vi "Get_DSC_Vals.vi"(8 "Machine":string, 9 "Shared Variable Control":refnum<k21>, 10 "Name":string, 11 "Authorization Header":T1[](array[typedef])) -> ()   [LabVIEW 2016]
uses:
  <vilib>/addons/_JKI.lib/REST Client/classes/REST Client/HTTP Header.ctl
  <vilib>/LVH/i3 JSON/JSON Parsing/Get Object Parameter Files/Get Object Parameter - Object.vi
  <vilib>/LVH/i3 JSON/JSON Parsing/Get Object Parameter Files/Get Object Parameter - String.vi
  <vilib>/addons/_JKI.lib/REST Client/classes/REST Client/REST Client.lvclass
  <vilib>/addons/_JKI.lib/Serialization/JSON/JKI JSON Serialization.lvlib
  <vilib>/LVH/i3 JSON/i3-json.lvlib
panel:
  in  "OK":bool
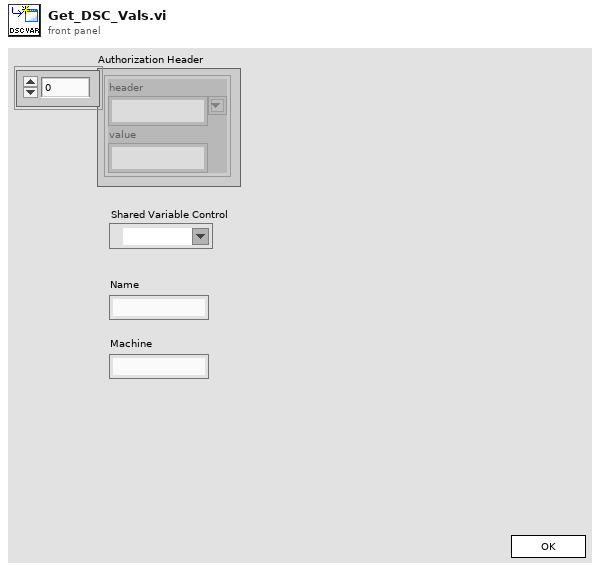
[diagram p1: front panel]
types:
  T1 = typedef "REST Client.lvlib/REST Client.lvclass/HTTP Header.ctl" = cluster{"header":string, "value":string}
  T2 = enum32{"Invalid", "Standard", "Closed", "Hidden", "Minimized", "Maximized"}
  T3 = enum32{"invalid app kind", "Development System", "Run Time System", "Student Edition", "Embedded LabVIEW", "Evaluation", "Custom"}
  T4 = cluster{"Core":cluster{"Current VI Reference":refnum<vi>, "Close Panel on Exit?":bool}, "New Reference":string, "Array of DSC References":cluster{string, string}[], "Authorization Header":T1[], "GID":string, "Name":string, "trimmed string":string, "Section GID":string}
  T5 = cluster{"Current VI Reference":refnum<vi>, "Close Panel on Exit?":bool}
  T6 = cluster{"data":cluster{"id":i32, "gid":string, "name":string, "resource_type":string}[]}
  T7 = cluster{"id":i32, "gid":string, "name":string, "resource_type":string}[]
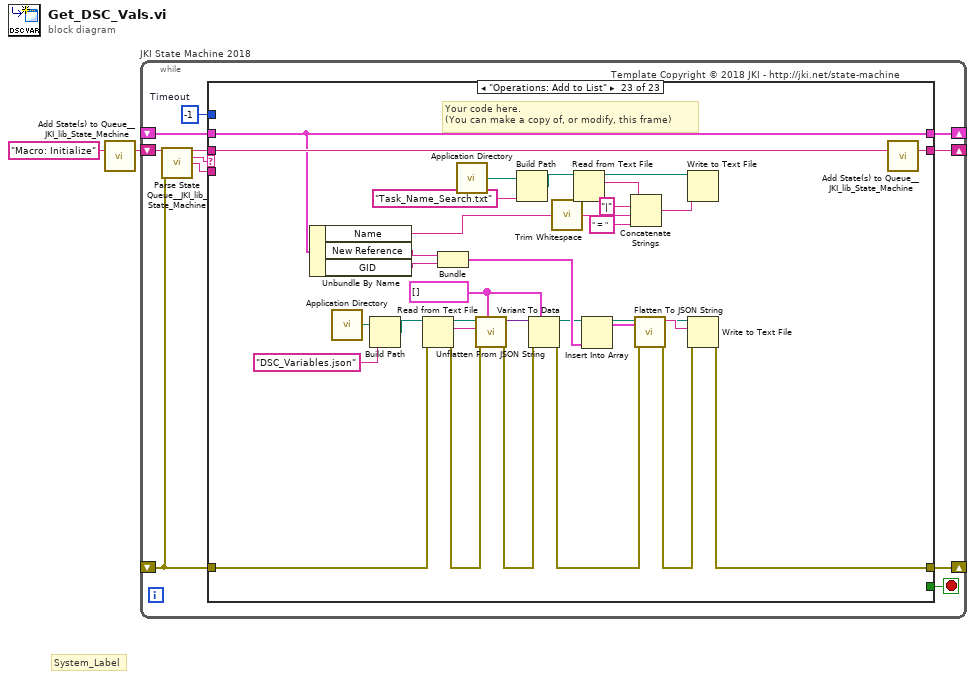
[diagram p0: block diagram]
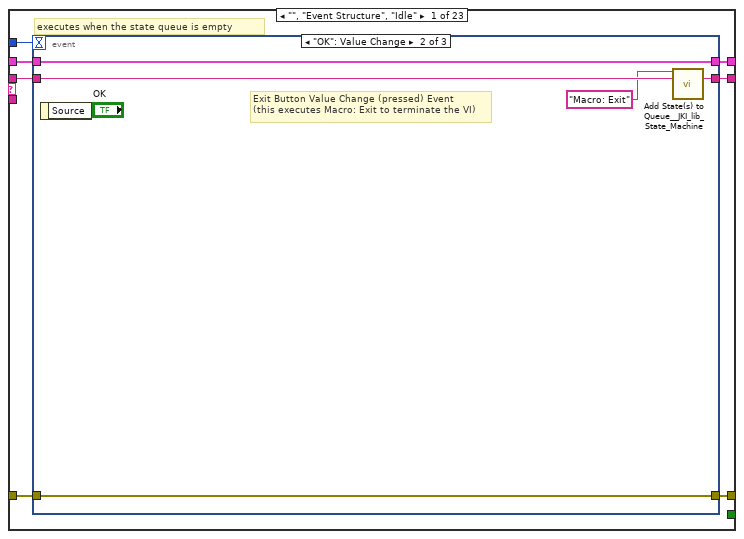
[diagram p2: hidden frame]
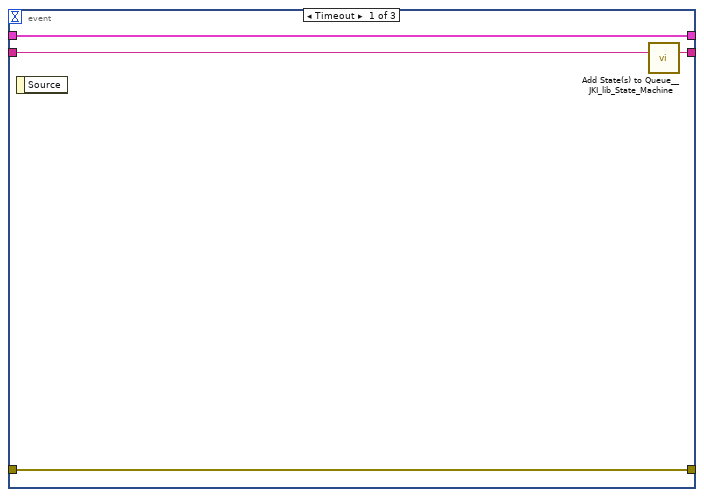
[diagram p3: hidden frame]
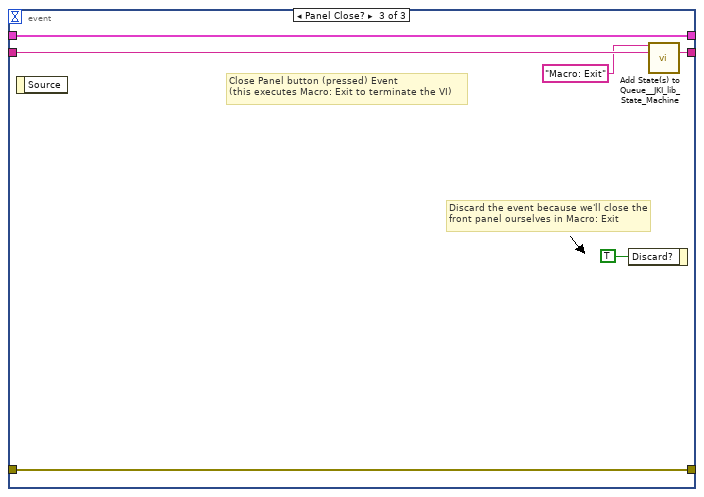
[diagram p4: hidden frame]
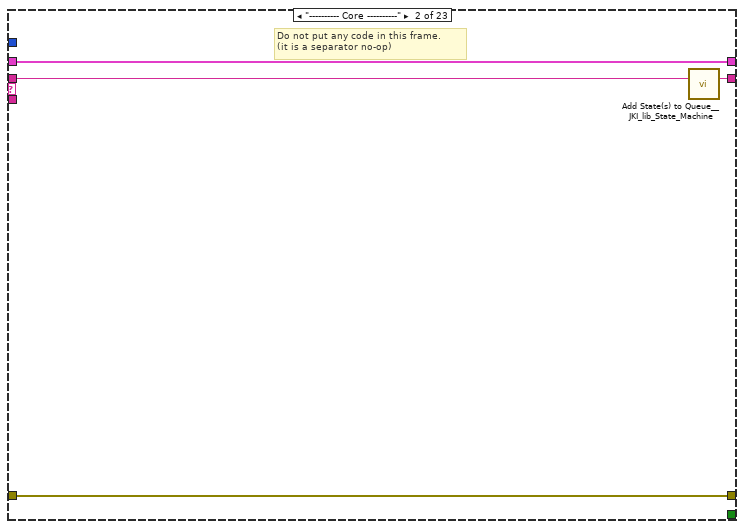
[diagram p5: hidden frame]
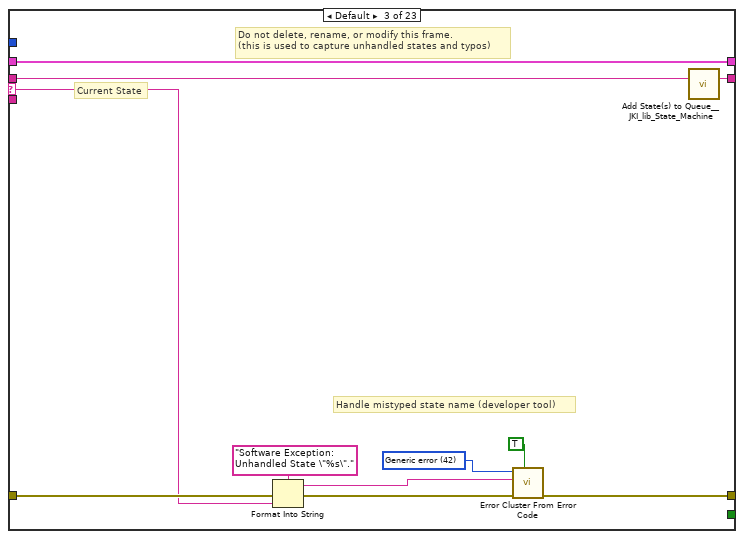
[diagram p6: hidden frame]
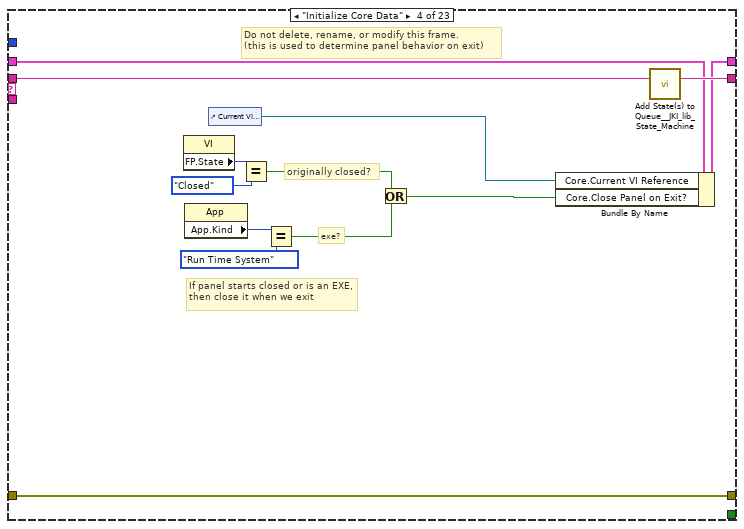
[diagram p7: hidden frame]
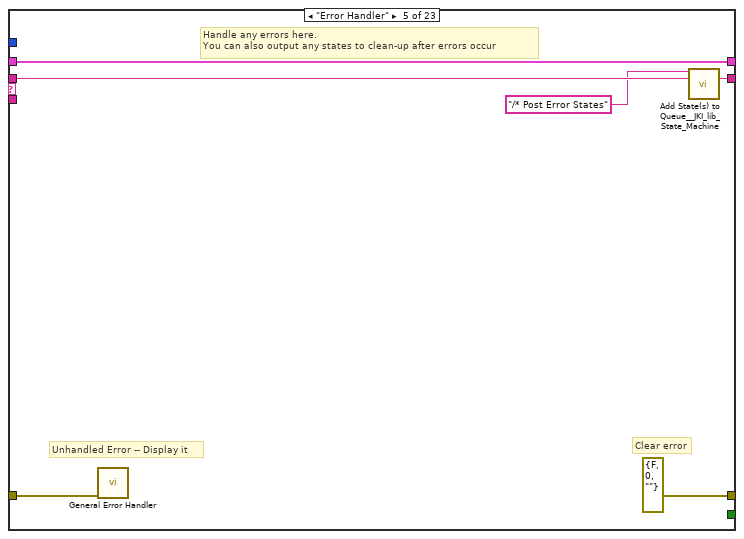
[diagram p8: hidden frame]
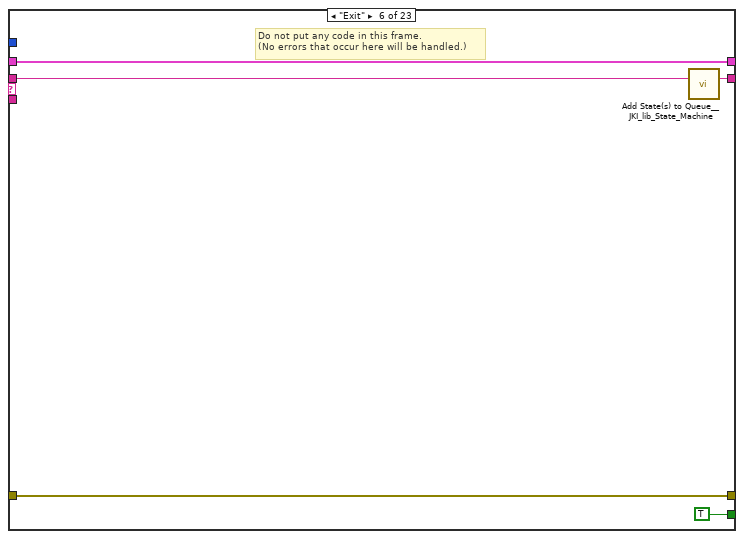
[diagram p9: hidden frame]
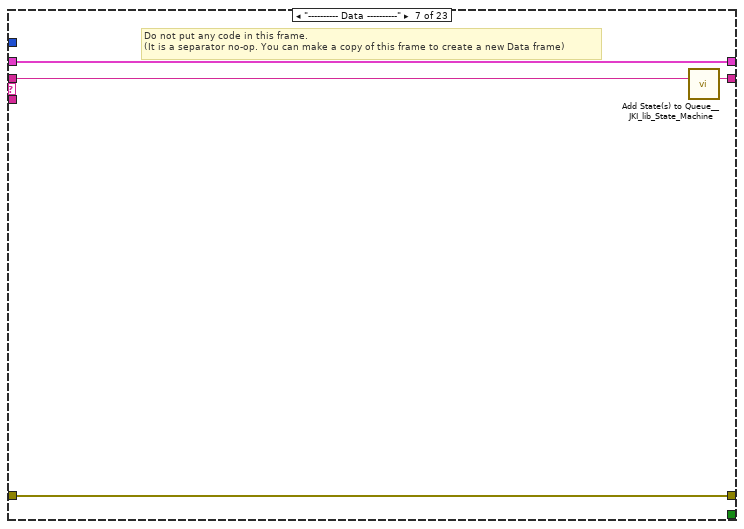
[diagram p10: hidden frame]
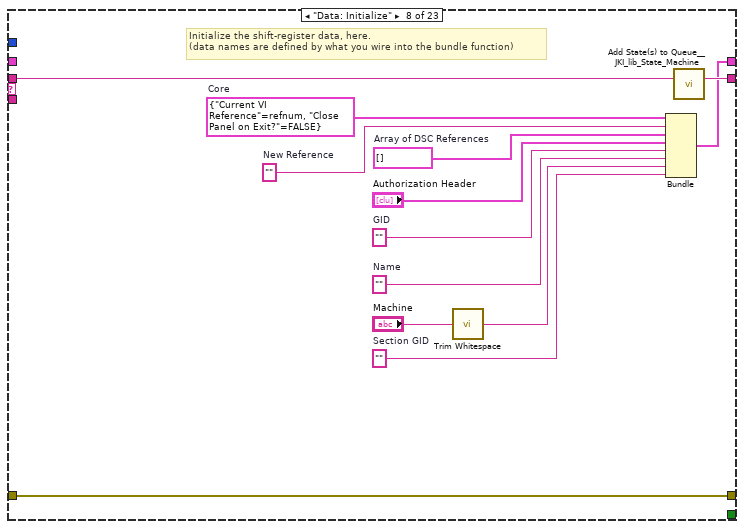
[diagram p11: hidden frame]
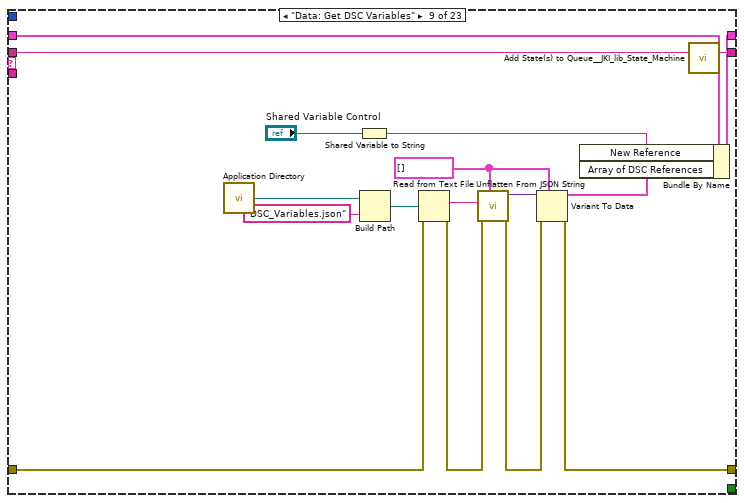
[diagram p12: hidden frame]
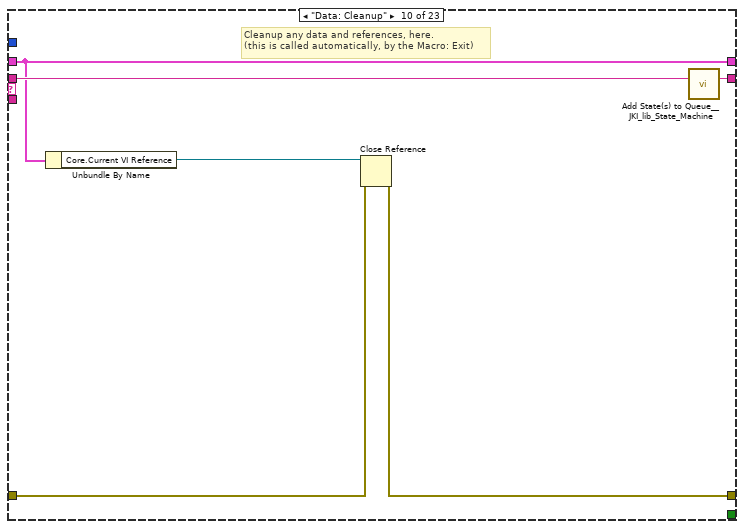
[diagram p13: hidden frame]
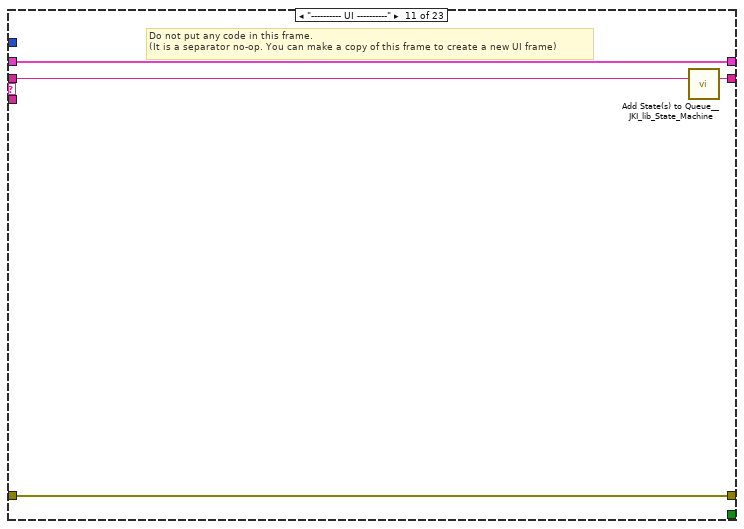
[diagram p14: hidden frame]
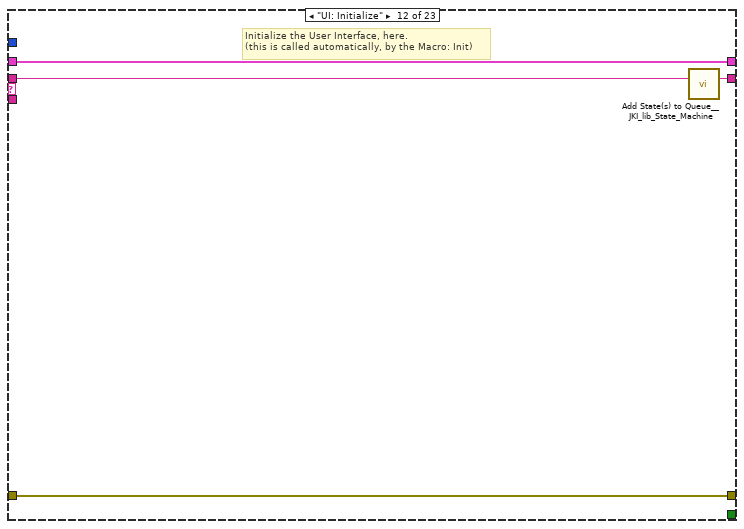
[diagram p15: hidden frame]
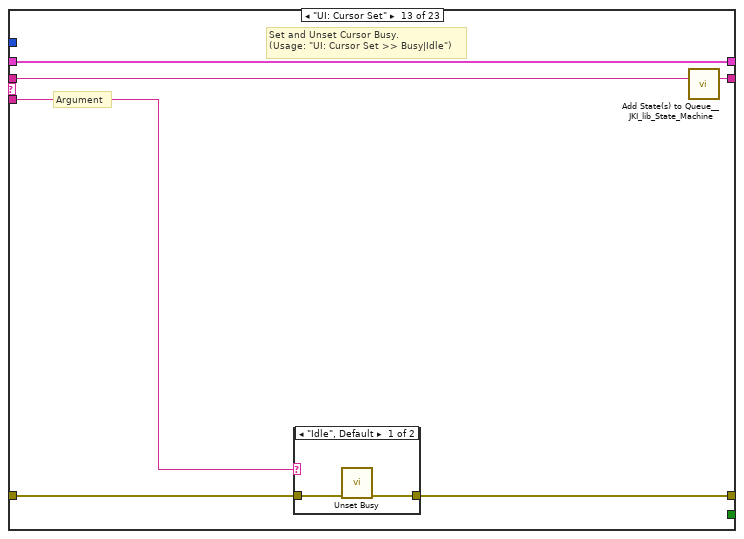
[diagram p16: hidden frame]
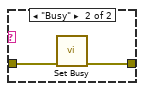
[diagram p17: hidden frame]
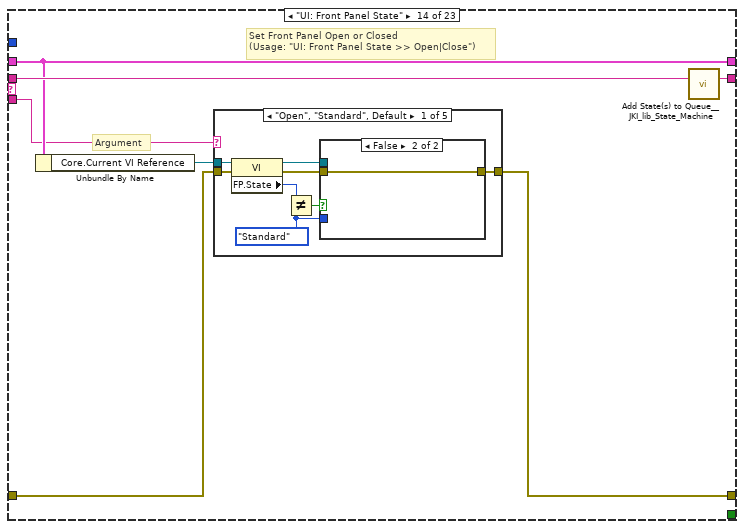
[diagram p18: hidden frame]
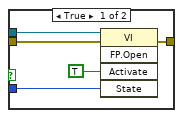
[diagram p19: hidden frame]
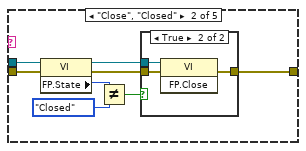
[diagram p20: hidden frame]
diagram:
  # "System_Label"
  n1 = call <vilib>:"Add State(s) to Queue__JKI_lib_State_Machine.vi"("State(s) in (\"\")"="Macro: Initialize") -> ("States Out"=w2:string)  [unwired: 14 in]
  n2 = while "JKI State Machine 2018" {
    shift-right: [w6] -> _
    shift-left: _ -> [w5]
    shift-right: [w9] -> _
    shift-left: _ -> [w3]
    shift-right: [w8] -> _
    shift-left: w2 -> [w10]
    stop <- w7 stop-if-true
    w4 = -1  # Timeout
    # "Template Copyright © 2018 JKI - http://jki.net/state-machine"
    n3 = call <vilib>:"Parse State Queue__JKI_lib_State_Machine.vi"("State Queue"=w10, "Error In (no error)"=w3) -> ("Remaining States"=w12:string, "Current State"=w13:string, "Arguments"=w11:string)  [unwired: 11 in]
    n4 = case shown="\"Operations: Add to List\"" w13 {
      selector: w13 -> [_ _ w40 _ _ _ _ _ _ _ _ _ _ _ _ _ _ _ _ _ _ _ _]
      tunnel: w12 -> [w20 w39 w44 w63 w69 w74 w78 w91 w108 w114 w118 w122 w128 w139 w208 w213 w223 w227 w237 w269 w307 w333 w363]
      tunnel: w11 -> [_ _ _ _ _ _ _ _ _ _ _ _ w123 w133 _ _ _ _ _ _ _ _ _]
      tunnel: w5 -> [w18 w36 w42 w56 w66 w72 w75 _ w105 w109 w115 w120 w126 w135 w205 w210 w220 w224 w234 w246 w301 w324 w361]
      tunnel: [w17 w37 w46 w60 errorcluster {"status"=FALSE, "code"=0, "source"=""} ("error out") w71 w76 w88 w96 w110 w116 w119 w124 w136 w206 w211 w221 w225 w235 w255 w296 w316 w357] -> w9
      tunnel: w3 -> [w16 w37 w45 w60 w65 w71 w76 w88 w95 w111 w116 w119 w125 w137 w206 w211 w221 w225 w235 w260 w299 w322 w358]
      tunnel: [w19 w38 w43 w62 w68 w73 w77 w90 w107 w113 w117 w121 w127 w138 w207 w212 w222 w226 w236 w268 w306 w332 w362] -> w8
      tunnel: [_ _ _ _ _ TRUE _ _ _ _ _ _ _ _ _ _ _ _ _ _ _ _ _] -> w7
      tunnel: [w15 w36 w42 w61 w66 w72 w75 w89 w104 w109 w115 w120 w126 w135 w205 w210 w220 w224 w234 w245 w300 w323 w361] -> w6
      tunnel: w4 -> [w14 _ _ _ _ _ _ _ _ _ _ _ _ _ _ _ _ _ _ _ _ _ _]
      frame "", "Event Structure", "Idle" {
        # "executes when the state queue is empty"
        n5 = event shown="[1] \"OK\": Value Change" {
          selector: _ -> [_ _ _]
          dyn-events: _ -> [_ _ _]
          timeout: w14 -> [_ _ _]
          tunnel: w20 -> [w24 w29 w35]
          tunnel: [w23 w28 w34] -> w19
          tunnel: w18 -> [w21 w26 w32]
          tunnel: [w22 w27 w33] -> w17
          tunnel: w16 -> [w22 w27 w33]
          tunnel: [w21 w26 w32] -> w15
          event Timeout {
            n6 = event-data() -> ()  [unwired: 1 in, 1 out]
            n7 = call <vilib>:"Add State(s) to Queue__JKI_lib_State_Machine.vi"("State(s) in (\"\")"=w24) -> ("States Out"=w23:string)  [unwired: 14 in]
          }
          event "OK": Value Change {
            # "Exit Button Value Change (pressed) Event\n(this executes Macro: Exit to terminate the VI)"
            n8 = event-data() -> ()  [unwired: 1 in, 1 out]
            n9 = call <vilib>:"Add State(s) to Queue__JKI_lib_State_Machine.vi"("State(s) in Front (\"\")"="Macro: Exit", "State(s) in (\"\")"=w29) -> ("States Out"=w28:string)  [unwired: 13 in]
          }
          event Panel Close? {
            # "Discard the event because we'll close the front panel ourselves in Macro: Exit"
            # "Close Panel button (pressed) Event\n(this executes Macro: Exit to terminate the VI)"
            n10 = event-data() -> ()  [unwired: 1 in, 1 out]
            n11 = event-data("Discard?"=TRUE) -> ()  [unwired: 1 in, 1 out]
            n12 = call <vilib>:"Add State(s) to Queue__JKI_lib_State_Machine.vi"("State(s) in Front (\"\")"="Macro: Exit", "State(s) in (\"\")"=w35) -> ("States Out"=w34:string)  [unwired: 13 in]
          }
        }
      }
      frame "---------- Core ----------" {
        # "Do not put any code in this frame.\n(it is a separator no-op)"
        n13 = call <vilib>:"Add State(s) to Queue__JKI_lib_State_Machine.vi"("State(s) in (\"\")"=w39) -> ("States Out"=w38:string)  [unwired: 14 in]
      }
      frame Default {
        w49 = 42 items=["No error", "Argument error", "Memory is full", "Out of zone", "End of file", "File already open", "Generic file I/O error", "File not found", "File permission error", "Disk is full", "Duplicate path", "Too many files open", "System feature not enabled", "Resource file not found", "Cannot add resource", "Resource not found", "Image not found", "Image memory error", "Pen does not exist", "Config type invalid", "Config token not found", "Config parse error", "Config memory error", "Bad external code format", "Bad external code offset", "External code not present", "Null window", "Destroy window error", "Null menu", "Print aborted", "Bad print record", "Print driver error", "Windows error during printing", "Memory error during printing", "Print dialog error", "Generic print error", "Invalid device refnum", "Device not found", "Device parameter error", "Device unit error", "Cannot open device", "Device call aborted", "Generic error", "Cancelled by user", "Object ID too low", "Object ID too high", "Object not in heap", "Unknown heap", "Unknown object (invalid DefProc)", "Unknown object (DefProc not in table)", "Message out of range", "Invalid (null) method", "Unknown message", "Manager call not supported", "Bad address", "Network operation in progress", "Network operation timed out", "Connection is busy", "Network attribute not supported", "Network error", "Address in use", "System out of memory", "Connection aborted", "Connection refused", "Not connected", "Already connected", "Connection closed", "Initialization error (interapplication manager)", "Bad occurrence", "Wait on unbound occurrence handler", "Occurrence queue overflow", "Datalog type conflict", "Unused", "Unrecognized type (interapplication manager)", "Memory corrupt", "Failed to make temporary DLL", "Old CIN version", "Drag socket not found", "Failed to load drop-object", "Failed to register OLE object", "Failed to release OLE object", "Format specifier type mismatch", "Unknown format specifier", "Too few format specifiers", "Too many format specifiers", "Scan failed", "Newer CIN version", "Error converting to variant", "Runtime menu error", "Password tampered", "Variant attribute not found", "Incompatible variant data type", "Event data is not available", "Event Store is not present", "Occurrence is not found", "Event Queue is not created", "Event info is not available", "Refnum passed is NULL", "Error retrieving Class GUID", "Error retrieving CoClass GUID", "Error retrieving TypeLib GUID.", "Bad built application magic bytes.", "Specific driver is different from the specific driver associated with the Logical Name.", "There is no session opened to the class driver.", "Max Error", "MAX - Error with config objects", "MAX - Error loading configuration", "MAX - Group not supported"]
        # "Current State"
        # "Do not delete, rename, or modify this frame.\n(this is used to capture unhandled states and typos)"
        # "Handle mistyped state name (developer tool)"
        n14 = Format Into String(format string="Software Exception: Unhandled State \"%s\"." ("message"), error in=w45, w40) -> (resulting string=w48:string, error out=w47:errorcluster)  [unwired: 1 in]
        n15 = call <vilib>:"Error Cluster From Error Code.vi"("show call chain? (False)"=TRUE, "error in (no error)"=w47, "error message (\"\")"=w48, "error code (0)"=w49) -> ("error out"=w46:errorcluster)  [unwired: 5 in]
        n16 = call <vilib>:"Add State(s) to Queue__JKI_lib_State_Machine.vi"("State(s) in (\"\")"=w44) -> ("States Out"=w43:string)  [unwired: 14 in]
      }
      frame "Initialize Core Data" {
        # "Do not delete, rename, or modify this frame.\n(this is used to determine panel behavior on exit)"
        # "originally closed?"
        # "exe?"
        # "If panel starts closed or is an EXE, then close it when we exit"
        n17 = property class="VI"() -> ("FP.State"=w53:T2)  [unwired: 2 in, 2 out]
        n18 = property class="App"() -> ("App.Kind"=w59:T3)  [unwired: 2 in, 2 out]
        n19 = control-ref of="Current VI Reference"() -> (w54:refnum<vi>)
        n20 = Equal?(x=w53, y=T2."Closed" ("Front Panel Window:State")) -> (x = y?=w51:bool)
        n21 = Equal?(x=w59, y=T3."Run Time System" ("Application:Kind")) -> (x = y?=w57:bool)
        n22 = Or(x=w51, y=w57) -> (x .or. y?=w55:bool)
        n23 = Bundle By Name(cluster=w56, "Core.Current VI Reference"=w54, "Core.Close Panel on Exit?"=w55) -> (w61:T4)
        n24 = call <vilib>:"Add State(s) to Queue__JKI_lib_State_Machine.vi"("State(s) in (\"\")"=w63) -> ("States Out"=w62:string)  [unwired: 14 in]
      }
      frame "Error Handler" {
        # "Unhandled Error -- Display it"
        # "Handle any errors here.\nYou can also output any states to clean-up after errors occur"
        # "Clear error"
        n25 = call <vilib>:"General Error Handler.vi"("error in (no error)"=w65) -> ()  [unwired: 10 in, 5 out]
        n26 = call <vilib>:"Add State(s) to Queue__JKI_lib_State_Machine.vi"("State(s) in Front (\"\")"="/* Post Error States", "State(s) in (\"\")"=w69) -> ("States Out"=w68:string)  [unwired: 13 in]
      }
      frame "Exit" {
        # "Do not put any code in this frame.\n(No errors that occur here will be handled.)"
        n27 = call <vilib>:"Add State(s) to Queue__JKI_lib_State_Machine.vi"("State(s) in (\"\")"=w74) -> ("States Out"=w73:string)  [unwired: 14 in]
      }
      frame "---------- Data ----------" {
        # "Do not put any code in this frame.\n(It is a separator no-op. You can make a copy of this frame to create a new Data frame)"
        n28 = call <vilib>:"Add State(s) to Queue__JKI_lib_State_Machine.vi"("State(s) in (\"\")"=w78) -> ("States Out"=w77:string)  [unwired: 14 in]
      }
      frame "Data: Initialize" {
        w79 = ""  # Section GID
        w82 = ""  # Name
        w83 = ""  # GID
        w85 = ""  # New Reference
        w86 = cluster{string, string}[] []  # Array of DSC References
        w87 = T5 {"Current VI Reference"=refnum, "Close Panel on Exit?"=FALSE}  # Core
        # "Initialize the shift-register data, here.\n(data names are defined by what you wire into the bundle function)"
        n29 = call <vilib>:"Trim Whitespace.vi"("string"="Machine") -> ("trimmed string"=w80:string)  [unwired: 1 in]
        n30 = Bundle("Core"=w87, "New Reference"=w85, "Array of DSC References"=w86, "Authorization Header"="Authorization Header", "GID"=w83, "Name"=w82, "trimmed string"=w80, "Section GID"=w79) -> (w89:T4)  [unwired: 1 in]
        n31 = call <vilib>:"Add State(s) to Queue__JKI_lib_State_Machine.vi"("State(s) in (\"\")"=w91) -> ("States Out"=w90:string)  [unwired: 14 in]
      }
      frame "Data: Get DSC Variables" {
        w92 = cluster{string, string}[] []
        n32 = call <vilib>:"Application Directory.vi"() -> ("Application Directory"=w101:path)
        n33 = Shared Variable to String(1:"Shared Variable Control") -> (0:w103:string)
        n34 = Build Path(base path=w101, name or relative path="DSC_Variables.json") -> (appended path=w100:path)
        n35 = Read from Text File(file (use dialog)=w100, error in=w95) -> (text=w97:string, error out=w94:errorcluster)  [unwired: 2 in, 2 out]
        n36 = call <vilib>:"Unflatten From JSON String.vi"("Type and Defaults"=w92, "error in (no error)"=w94, "JSON String"=w97) -> ("error out"=w93:errorcluster, "Variant"=w99:variant)  [unwired: 7 in]
        n37 = Variant To Data(error in=w93, type=w92, Variant=w99) -> (data=w98:cluster{string, string}[], error out=w96:errorcluster)
        n38 = Bundle By Name(cluster=w105, "New Reference"=w103, "Array of DSC References"=w98) -> (w104:T4)
        n39 = call <vilib>:"Add State(s) to Queue__JKI_lib_State_Machine.vi"("State(s) in (\"\")"=w108) -> ("States Out"=w107:string)  [unwired: 14 in]
      }
      frame "Data: Cleanup" {
        # "Cleanup any data and references, here.\n(this is called automatically, by the Macro: Exit)"
        n40 = Unbundle By Name(w109) -> ("Core.Current VI Reference"=w112:refnum<vi>)
        n41 = Close Reference(reference=w112, error in (no error)=w111) -> (error out=w110:errorcluster)
        n42 = call <vilib>:"Add State(s) to Queue__JKI_lib_State_Machine.vi"("State(s) in (\"\")"=w114) -> ("States Out"=w113:string)  [unwired: 14 in]
      }
      frame "---------- UI ----------" {
        # "Do not put any code in this frame.\n(It is a separator no-op. You can make a copy of this frame to create a new UI frame)"
        n43 = call <vilib>:"Add State(s) to Queue__JKI_lib_State_Machine.vi"("State(s) in (\"\")"=w118) -> ("States Out"=w117:string)  [unwired: 14 in]
      }
      frame "UI: Initialize" {
        # "Initialize the User Interface, here.\n(this is called automatically, by the Macro: Init)"
        n44 = call <vilib>:"Add State(s) to Queue__JKI_lib_State_Machine.vi"("State(s) in (\"\")"=w122) -> ("States Out"=w121:string)  [unwired: 14 in]
      }
      frame "UI: Cursor Set" {
        # "Argument"
        # "Set and Unset Cursor Busy.\n(Usage: \"UI: Cursor Set >> Busy|Idle\")"
        n45 = case shown="\"Idle\", Default" w123 {
          tunnel: w125 -> [w130 w132]
          tunnel: [w129 w131] -> w124
          frame "Idle", Default {
            n46 = call <vilib>:"Unset Busy.vi"("error in (no error)"=w130) -> ("error out"=w129:errorcluster)  [unwired: 10 in]
          }
          frame "Busy" {
            n47 = call <vilib>:"Set Busy.vi"("error in (no error)"=w132) -> ("error out"=w131:errorcluster)  [unwired: 9 in, 1 out]
          }
        }
        n48 = call <vilib>:"Add State(s) to Queue__JKI_lib_State_Machine.vi"("State(s) in (\"\")"=w128) -> ("States Out"=w127:string)  [unwired: 14 in]
      }
      frame "UI: Front Panel State" {
        # "Argument"
        # "Set Front Panel Open or Closed\n(Usage: \"UI: Front Panel State >> Open|Close\")"
        n49 = Unbundle By Name(w135) -> ("Core.Current VI Reference"=w134:refnum<vi>)
        n50 = case shown="\"Open\", \"Standard\", Default" w133 {
          tunnel: w137 -> [w145 w160 w171 w184 w197]
          tunnel: [w147 w161 w173 w186 w199] -> w136
          tunnel: w134 -> [w146 w158 w172 w185 w198]
          frame "Open", "Standard", Default {
            w140 = T2."Standard" ("State")
            n51 = property class="VI"(reference=w146, error in=w145) -> (reference out=w143:refnum<vi>, error out=w144:errorcluster, "FP.State"=w142:T2)
            n52 = Not Equal?(x=w142, y=w140) -> (x != y?=w141:bool)
            n53 = case shown="False" w141 {
              tunnel: [w151 w153] -> w147
              tunnel: w144 -> [w150 w153]
              tunnel: w143 -> [w149 _]
              tunnel: w140 -> [w148 _]
              frame True {
                n54 = invoke class="VI" method="FP.Open"(reference=w149, error in=w150, "Activate"=TRUE, "State"=w148) -> (error out=w151:errorcluster)  [unwired: 1 in, 4 out]
              }
              frame False {
              }
            }
          }
          frame "Close", "Closed" {
            n55 = property class="VI"(reference=w158, error in=w160) -> (reference out=w157:refnum<vi>, error out=w159:errorcluster, "FP.State"=w155:T2)
            n56 = Not Equal?(x=w155, y=T2."Closed" ("Front Panel Window:State")) -> (x != y?=w154:bool)
            n57 = case shown="True" w154 {
              tunnel: [w162 w165] -> w161
              tunnel: w159 -> [w162 w164]
              tunnel: w157 -> [_ w163]
              frame False {
              }
              frame True {
                n58 = invoke class="VI" method="FP.Close"(reference=w163, error in=w164) -> (error out=w165:errorcluster)  [unwired: 1 in, 2 out]
              }
            }
          }
          frame "Hidden", "Hide" {
            w166 = T2."Hidden" ("State")
            n59 = property class="VI"(reference=w172, error in=w171) -> (reference out=w169:refnum<vi>, error out=w170:errorcluster, "FP.State"=w168:T2)
            n60 = Not Equal?(x=w168, y=w166) -> (x != y?=w167:bool)
            n61 = case shown="True" w167 {
              tunnel: [w177 w178] -> w173
              tunnel: w170 -> [w176 w178]
              tunnel: w169 -> [w175 _]
              tunnel: w166 -> [w174 _]
              frame True {
                n62 = invoke class="VI" method="FP.Open"(reference=w175, error in=w176, "State"=w174) -> (error out=w177:errorcluster)  [unwired: 2 in, 4 out]
              }
              frame False {
              }
            }
          }
          frame "Minimize", "Minimized" {
            w179 = T2."Minimized" ("State")
            n63 = property class="VI"(reference=w185, error in=w184) -> (reference out=w182:refnum<vi>, error out=w183:errorcluster, "FP.State"=w181:T2)
            n64 = Not Equal?(x=w181, y=w179) -> (x != y?=w180:bool)
            n65 = case shown="True" w180 {
              tunnel: [w190 w191] -> w186
              tunnel: w183 -> [w189 w191]
              tunnel: w182 -> [w188 _]
              tunnel: w179 -> [w187 _]
              frame True {
                n66 = invoke class="VI" method="FP.Open"(reference=w188, error in=w189, "State"=w187) -> (error out=w190:errorcluster)  [unwired: 2 in, 4 out]
              }
              frame False {
              }
            }
          }
          frame "Maximize", "Maximized" {
            w192 = T2."Maximized" ("State")
            n67 = property class="VI"(reference=w198, error in=w197) -> (reference out=w195:refnum<vi>, error out=w196:errorcluster, "FP.State"=w194:T2)
            n68 = Not Equal?(x=w194, y=w192) -> (x != y?=w193:bool)
            n69 = case shown="True" w193 {
              tunnel: [w203 w204] -> w199
              tunnel: w196 -> [w202 w204]
              tunnel: w195 -> [w201 _]
              tunnel: w192 -> [w200 _]
              frame True {
                n70 = invoke class="VI" method="FP.Open"(reference=w201, error in=w202, "State"=w200) -> (error out=w203:errorcluster)  [unwired: 2 in, 4 out]
              }
              frame False {
              }
            }
          }
        }
        n71 = call <vilib>:"Add State(s) to Queue__JKI_lib_State_Machine.vi"("State(s) in (\"\")"=w139) -> ("States Out"=w138:string)  [unwired: 14 in]
      }
      frame "---------- Macro ----------" {
        # "Do not put any code in this frame.\n(It is a separator no-op. You can make a copy of this frame to create a new Macro frame)"
        n72 = call <vilib>:"Add State(s) to Queue__JKI_lib_State_Machine.vi"("State(s) in (\"\")"=w208) -> ("States Out"=w207:string)  [unwired: 14 in]
      }
      frame "Macro: Initialize" {
        # "Initialization Macro\n(This is called once, when the VI starts)"
        n73 = call <vilib>:"Add State(s) to Queue__JKI_lib_State_Machine.vi"("State(s) in Front (\"\")"="Data: Initialize\nInitialize Core Data\nUI: Initialize\nUI: Front Panel State >> Open\nData: Get DSC Variables\nOperations: Check List", "State(s) in (\"\")"=w213) -> ("States Out"=w212:string)  [unwired: 13 in]
      }
      frame "Macro: Exit" {
        # "Exit Macro\n(This is called once, when the VI exits)"
        n74 = Unbundle By Name(w220) -> ("Core.Close Panel on Exit?"=w219:bool)
        n75 = Select(t="UI: Front Panel State >> Close", s=w219, f="") -> (s? t:f=w216:string)
        n76 = call <vilib>:"Add State(s) to Queue__JKI_lib_State_Machine.vi"("State(s) in (\"\")"=w216, "State(s) at Back (\"\")"="Data: Cleanup\nExit") -> ("States Out"=w214:string)  [unwired: 13 in]
        n77 = call <vilib>:"Add State(s) to Queue__JKI_lib_State_Machine.vi"("State(s) in Front (\"\")"=w214, "State(s) in (\"\")"=w223) -> ("States Out"=w222:string)  [unwired: 13 in]
      }
      frame "---------- Operations ----------" {
        # "Template Separator\n(You can make a copy of, or modify, this frame)"
        n78 = call <vilib>:"Add State(s) to Queue__JKI_lib_State_Machine.vi"("State(s) in (\"\")"=w227) -> ("States Out"=w226:string)  [unwired: 14 in]
      }
      frame "Operations: Check List" {
        # "Your code here.\n(You can make a copy of, or modify, this frame)"
        n79 = Unbundle By Name(w234) -> ("Array of DSC References"=w233:cluster{string, string}[], "New Reference"=w232:string)
        n80 = for {
          tunnel: w233 -> [w242] mode=indexing
          tunnel: w232 -> [w241]
          tunnel: [w240] -> w230 mode=indexing
          stop <- w240 stop-if-true
          n81 = Unbundle(w242) -> (w243:string)  [unwired: 1 out]
          n82 = Equal?(x=w243, y=w241) -> (x = y?=w240:bool)
        }
        n83 = Search 1D Array(1D array=w230, element=TRUE) -> (index of element=w228:i32)  [unwired: 1 in]
        n84 = case shown="-1" w228 {
          tunnel: ["Macro: Exit" "Operations: Check Section\nOperations: Make Asana Task\nOperations: Add to List"] -> w231
          frame 0, Default {
            n85 = call "Display Message to User"() -> ()  [unwired: 10 in, 2 out]
          }
          frame -1 {
          }
        }
        n86 = call <vilib>:"Add State(s) to Queue__JKI_lib_State_Machine.vi"("State(s) in Front (\"\")"=w231, "State(s) in (\"\")"=w237) -> ("States Out"=w236:string)  [unwired: 13 in]
      }
      frame "Operations: Check Section" {
        w262 = T6 {"data"=[]}
        # "Your code here.\n(You can make a copy of, or modify, this frame)"
        n87 = Unbundle By Name(w246) -> ("Authorization Header"=w254:T1[], "trimmed string"=w249:string)
        n88 = call <vilib>:"Create REST Client.vi"("error in (no error)"=w260, "Base URL"="https://app.asana.com/api/1.0") -> ("error out"=w259:errorcluster, "REST Client out"=w267:refnum<class "REST Client.lvclass">)  [unwired: 8 in]
        n89 = call-dynamic "HTTP GET.vi"("request specific headers"=w254, "error in (no error)"=w259, "Path"="/projects/1122243734894450/sections", "REST Client in"=w267) -> ("error out"=w258:errorcluster, "Response body"=w261:string, "REST Client out"=w266:refnum<class "REST Client.lvclass">)  [unwired: 2 in, 3 out]
        n90 = call-dynamic "Destroy REST Client.vi"("error in (no error)"=w258, "REST Client in"=w266) -> ("error out"=w257:errorcluster)  [unwired: 9 in]
        n91 = call <vilib>:"Unflatten From JSON String.vi"("Type and Defaults"=w262, "error in (no error)"=w257, "JSON String"=w261) -> ("error out"=w256:errorcluster, "Variant"=w263:variant)  [unwired: 7 in]
        n92 = Variant To Data(error in=w256, type=w262, Variant=w263) -> (data=w253:T6, error out=w255:errorcluster)
        n93 = Unbundle(w253) -> ("data"=w252:T7)
        n94 = for {
          tunnel: w252 -> [w278] mode=indexing
          tunnel: [w277] -> w251 mode=indexing
          tunnel: [w276] -> w247 mode=indexing
          n95 = Unbundle By Name(w278) -> ("gid"=w276:string, "name"=w277:string)
        }
        n96 = Search 1D Array(1D array=w251, element=w249) -> (index of element=w250:i32)  [unwired: 1 in]
        n97 = case shown="-1" w250 {
          selector: w250 -> [w272 _]
          tunnel: ["" "Operations: Make Section"] -> w248
          tunnel: w247 -> [w273 _]
          tunnel: [w271 ""] -> w244
          frame 0, Default {
            n98 = Index Array(array=w273, index=w272) -> (element=w271:string)
          }
          frame -1 {
          }
        }
        n99 = Bundle By Name(cluster=w246, "Section GID"=w244) -> (w245:T4)
        n100 = call <vilib>:"Add State(s) to Queue__JKI_lib_State_Machine.vi"("State(s) in Front (\"\")"=w248, "State(s) in (\"\")"=w269) -> ("States Out"=w268:string)  [unwired: 13 in]
      }
      frame "Operations: Make Asana Task" {
        n101 = Unbundle By Name(w301) -> ("Section GID"=w291:string, "Authorization Header"=w295:T1[])
        n102 = Concatenate Strings("{\"data\": { \"name\":  \"" ("Request body"), "Name", " = \", \"projects\": \"1122243734894450\", \"memberships\": [{\"project\": \"1122243734894450\", \"section\": \"", w291, "\"}]}}" ("string")) -> (w294:string)
        n103 = call <vilib>:"Create REST Client.vi"("error in (no error)"=w299, "Base URL"="https://app.asana.com/api/1.0") -> ("error out"=w298:errorcluster, "REST Client out"=w305:refnum<class "REST Client.lvclass">)  [unwired: 8 in]
        n104 = call-dynamic "HTTP POST.vi"("request specific headers"=w295, "error in (no error)"=w298, "Request body"=w294, "Path"="/tasks", "REST Client in"=w305) -> ("error out"=w280:errorcluster, "Response body"=w284:string, "REST Client out"=w292:refnum<class "REST Client.lvclass">)  [unwired: 1 in, 3 out]
        n105 = call <vilib>:"Parse JSON.vi"("error in (no error)"=w280, "JSON String"=w284) -> ("error out"=w281:errorcluster, "JSON Tree"=w288:variant)  [unwired: 6 in, 2 out]
        n106 = call-poly <vilib>:"Get Object Parameter.vi"("error in (no error)"=w281, "Parameter Name"="data", "JSON Tree In (JSON Object)"=w288) -> ("error out"=w282:errorcluster, "JSON Object"=w287:variant)  [unwired: 5 in, 2 out]
        n107 = call-poly <vilib>:"Get Object Parameter.vi"("error in (no error)"=w282, "Parameter Name"="gid", "JSON Tree In (JSON Object)"=w287) -> ("error out"=w283:errorcluster, "String Value"=w279:string)  [unwired: 5 in, 2 out]
        n108 = Bundle By Name(cluster=w301, "GID"=w279, "Name"="Name") -> (w300:T4)
        n109 = call-dynamic "Destroy REST Client.vi"("error in (no error)"=w283, "REST Client in"=w292) -> ("error out"=w296:errorcluster)  [unwired: 9 in]
        n110 = call <vilib>:"Add State(s) to Queue__JKI_lib_State_Machine.vi"("State(s) in (\"\")"=w307, "State(s) at Back (\"\")"="Macro: Exit" ("State(s) in Front (\"\")")) -> ("States Out"=w306:string)  [unwired: 13 in]
      }
      frame "Operations: Make Section" {
        n111 = Unbundle By Name(w324) -> ("trimmed string"=w318:string, "Authorization Header"=w329:T1[])
        n112 = Concatenate Strings("{\"data\": {\"name\":  \"" ("Request body"), w318, "\"}}") -> (w325:string)
        n113 = call <vilib>:"Create REST Client.vi"("error in (no error)"=w322, "Base URL"="https://app.asana.com/api/1.0") -> ("error out"=w320:errorcluster, "REST Client out"=w331:refnum<class "REST Client.lvclass">)  [unwired: 8 in]
        n114 = call-dynamic "HTTP POST.vi"("request specific headers"=w329, "error in (no error)"=w320, "Request body"=w325, "Path"="/projects/1122243734894450/sections", "REST Client in"=w331) -> ("error out"=w321:errorcluster, "Response body"=w313:string, "REST Client out"=w330:refnum<class "REST Client.lvclass">)  [unwired: 1 in, 3 out]
        n115 = call-dynamic "Destroy REST Client.vi"("error in (no error)"=w321, "REST Client in"=w330) -> ("error out"=w317:errorcluster)  [unwired: 9 in]
        n116 = call <vilib>:"Parse JSON.vi"("error in (no error)"=w317, "JSON String"=w313) -> ("error out"=w314:errorcluster, "JSON Tree"=w312:variant)  [unwired: 6 in, 2 out]
        n117 = call-poly <vilib>:"Get Object Parameter.vi"("error in (no error)"=w314, "Parameter Name"="data", "JSON Tree In (JSON Object)"=w312) -> ("error out"=w315:errorcluster, "JSON Object"=w311:variant)  [unwired: 5 in, 2 out]
        n118 = call-poly <vilib>:"Get Object Parameter.vi"("error in (no error)"=w315, "Parameter Name"="gid", "JSON Tree In (JSON Object)"=w311) -> ("error out"=w316:errorcluster, "String Value"=w308:string)  [unwired: 5 in, 2 out]
        n119 = Bundle By Name(cluster=w324, "Section GID"=w308) -> (w323:T4)
        n120 = call <vilib>:"Add State(s) to Queue__JKI_lib_State_Machine.vi"("State(s) in (\"\")"=w333) -> ("States Out"=w332:string)  [unwired: 14 in]
      }
      frame "Operations: Add to List" {
        w338 = cluster{string, string}[] []
        # "Your code here.\n(You can make a copy of, or modify, this frame)"
        n121 = Unbundle By Name(w361) -> ("Name"=w336:string, "New Reference"=w347:string, "GID"=w346:string)
        n122 = call <vilib>:"Application Directory.vi"() -> ("Application Directory"=w356:path)
        n123 = Build Path(base path=w356, name or relative path="DSC_Variables.json") -> (appended path=w337:path)
        n124 = Read from Text File(file (use dialog)=w337, error in=w358) -> (text=w355:string, error out=w354:errorcluster)  [unwired: 2 in, 2 out]
        n125 = Bundle("New Reference"=w347, "GID"=w346) -> (w359:cluster{"New Reference":string, "GID":string})  [unwired: 1 in]
        n126 = call <vilib>:"Application Directory.vi"() -> ("Application Directory"=w345:path)
        n127 = call <vilib>:"Unflatten From JSON String.vi"("Type and Defaults"=w338, "error in (no error)"=w354, "JSON String"=w355) -> ("error out"=w349:errorcluster, "Variant"=w353:variant)  [unwired: 7 in]
        n128 = Build Path(base path=w345, name or relative path="Task_Name_Search.txt") -> (appended path=w339:path)
        n129 = Variant To Data(error in=w349, type=w338, Variant=w353) -> (data=w334:cluster{string, string}[], error out=w348:errorcluster)
        n130 = call <vilib>:"Trim Whitespace.vi"("string"=w336) -> ("trimmed string"=w335:string)  [unwired: 1 in]
        n131 = Read from Text File(file (use dialog)=w339) -> (text=w343:string)  [unwired: 3 in, 3 out]
        n132 = Insert Into Array(array=w334, new element=w359) -> (w352:cluster{string, string}[])  [unwired: 1 in]
        n133 = Concatenate Strings(w343, "|" ("string"), w335, " = " ("string")) -> (w340:string)
        n134 = call <vilib>:"Flatten To JSON String.vi"("error in (no error)"=w348, "Variant"=w352) -> ("error out"=w351:errorcluster, "JSON String"=w350:string)  [unwired: 8 in]
        n135 = Write to Text File(file (use dialog)=w339, text=w340) -> ()  [unwired: 2 in, 3 out]
        n136 = Write to Text File(file (use dialog)=w337, text=w350, error in=w351) -> (error out=w357:errorcluster)  [unwired: 1 in, 2 out]
        n137 = call <vilib>:"Add State(s) to Queue__JKI_lib_State_Machine.vi"("State(s) in (\"\")"=w363) -> ("States Out"=w362:string)  [unwired: 14 in]
      }
    }
  }
